vi "VI_origin.vi"(3 "VI":refnum<vi>) -> (1 "Origin":T1)   [LabVIEW 2015]
uses:
  <vilib>/Utility/miscctls.llb/LVPointTypeDef.ctl
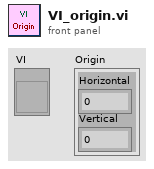
[diagram p1: front panel]
types:
  T1 = typedef "LVPointTypeDef.ctl" = cluster{"Horizontal":i16, "Vertical":i16}
  T2 = typedef "LVRectTypeDef.ctl" = cluster{"Left":i16, "Top":i16, "Right":i16, "Bottom":i16}
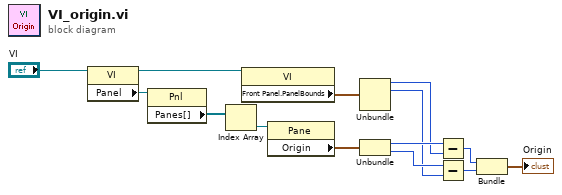
[diagram p0: block diagram]
diagram:
  n1 = property class="VI"(reference="VI") -> (reference out=w11:refnum<vi>, "Panel"=w13:refnum<vi>)  [unwired: 1 in, 1 out]
  n2 = property class="Pnl"(reference=w13) -> ("Panes[]"=w12:refnum<vi>[])  [unwired: 1 in, 2 out]
  n3 = Index Array(array=w12) -> (element=w14:refnum<vi>)  [unwired: 1 in]
  n4 = property class="VI"(reference=w11) -> ("Front Panel.PanelBounds"=w10:T2)  [unwired: 1 in, 2 out]
  n5 = property class="Pane"(reference=w14) -> ("Origin"=w9:T1)  [unwired: 1 in, 2 out]
  n6 = Unbundle(w10) -> ("Left"=w6:i16, "Top"=w4:i16)  [unwired: 2 out]
  n7 = Unbundle(w9) -> ("Horizontal"=w7:i16, "Vertical"=w5:i16)
  n8 = Subtract(x=w7, y=w6) -> (x-y=w3:i16)
  n9 = Subtract(x=w5, y=w4) -> (x-y=w2:i16)
  n10 = Bundle(w3, w2) -> (→"Origin":cluster{i16, i16})  [unwired: 1 in]
